vi "题目3温度测量子VI.vi"() -> ()   [LabVIEW 2017]
panel:
  out "温度":string
  in  "温度单位":bool
  in  "停止":bool
  out "温度计":dbl(slide) scale=0.0..210.0
  # "℃"
  # "℉"
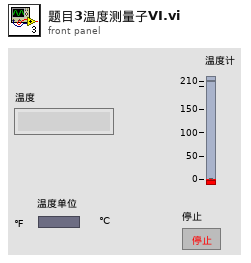
[diagram p1: front panel]
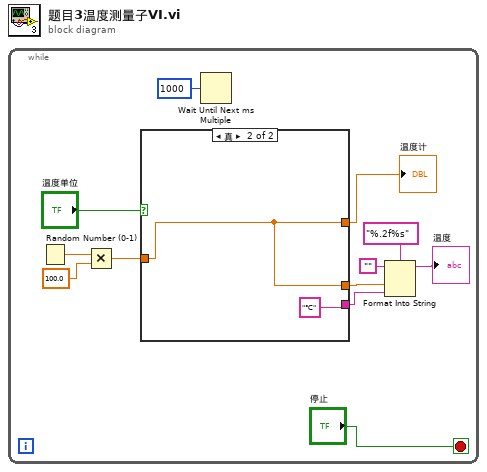
[diagram p0: block diagram]
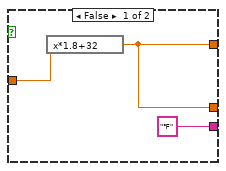
[diagram p2: hidden frame]
diagram:
  n1 = while {
    stop <- "停止" stop-if-true
    n2 = Random Number (0-1)() -> (number: 0 to 1=w12:dbl)
    n3 = Multiply(x=w12, y=100.0) -> (x*y=w9:dbl)
    n4 = case shown="真" "温度单位" {
      tunnel: w9 -> [w15 w17]
      tunnel: [w13 w17] -> w1
      tunnel: [w13 w17] -> w4
      tunnel: ["℉" "℃"] -> w3
      frame False {
        n5 = expression code="x*1.8+32"(w15) -> (w13:dbl)
      }
      frame True {
      }
    }
    "温度计" <- w1
    n6 = Wait Until Next ms Multiple(millisecond multiple=u32 1000 ("毫秒倍数")) -> ()  [unwired: 1 out]
    n7 = Format Into String(format string="%.2f%s" ("格式字符串"), initial string="" ("初始字符串"), w4, w3) -> (resulting string=→"温度":string)  [unwired: 1 in, 1 out]
  }
